vi "Set data.vi"(8 "error in (no error)":errorcluster caption="entrée d'erreur (pas d'erreur)", 10 "data":waveform(dbl)[](array[waveform]) caption="Data Read", 11 "Class Ana (Default) en entrée":refnum<class "Class Ana (Default).lvclass">) -> (0 "error out":errorcluster caption="sortie d'erreur", 3 "Class Ana (Default) en sortie":refnum<class "Class Ana (Default).lvclass">)   [LabVIEW 2020, in "Library Instrument & Equipement.lvlib" / "Library Ana.lvlib" / "Class Ana (Default).lvclass"]
uses:
  Class Ana (Default).lvclass
  Class Ana (Default).lvclass/Class Ana (Default).ctl
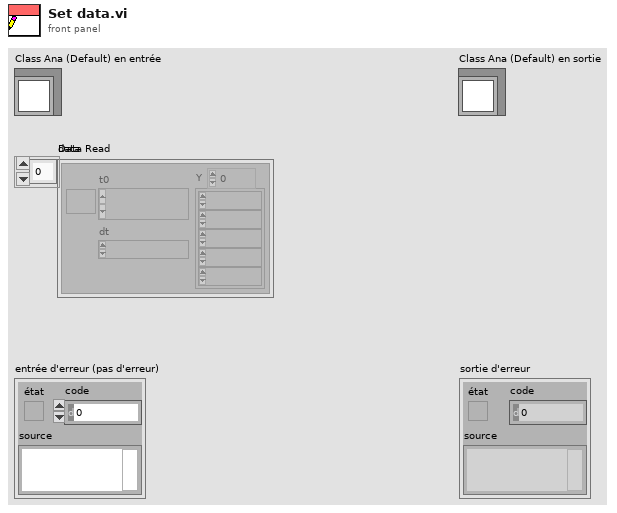
[diagram p1: front panel]
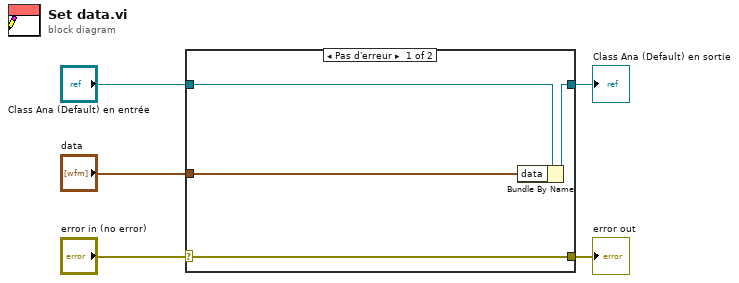
[diagram p0: block diagram]
diagram:
  n1 = case shown="Pas d'erreur" "error in (no error)" {
    selector: "error in (no error)" -> [w9 w10]
    tunnel: [w9 w10] -> w4
    tunnel: [w7 w11] -> w2
    tunnel: "Class Ana (Default) en entrée" -> [w8 w11]
    tunnel: "data" -> [w6 _]
    frame No Error {
      n2 = Bundle By Name(cluster=w8, "data"=w6) -> (w7:refnum<class "Class Ana (Default).lvclass">)
    }
    frame Error {
    }
  }
  "error out" <- w4
  "Class Ana (Default) en sortie" <- w2
